vi "Load data into Tree.vi"(8 "error in (no error)":errorcluster, 11 "Execution UI In":refnum<class "Execution UI.lvclass">) -> (0 "error out":errorcluster, 3 "Execution UI Out":refnum<class "Execution UI.lvclass">)   [LabVIEW 2020, in "Execution UI.lvclass"]
uses:
  Execution UI.lvclass
  Execution UI.lvclass/Execution UI.ctl
  Helper Classes/Test Finder/Test Finder.lvclass/Test Finder.ctl
  Helper Classes/Result Table/Result Table/Result Table.lvclass/Result Table.ctl
  Helper Classes/Test Result Tree/Test Result Tree.lvclass
  C:/Users/anton/Documents/GitHub/LUnit/source/Framework/Helper Classes/Test Tree/Test Tree.lvclass
  Helper Classes/Test Finder/Public/Accessors/Read Test Method Names.vi
  Helper Classes/Test Tree/Test Tree.lvclass
  Helper Classes/Test Finder/Test Finder.lvclass
  Helper Classes/Result Table/Result Table/Result Table.lvclass
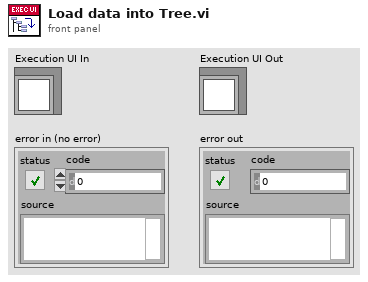
[diagram p1: front panel]
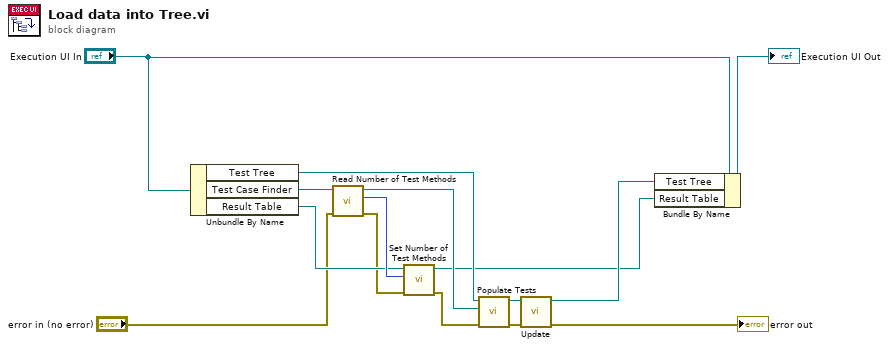
[diagram p0: block diagram]
diagram:
  n1 = Unbundle By Name("Execution UI In") -> ("Test Tree"=w11:refnum<class "Test Result Tree.lvclass">, "Test Case Finder"=w8:refnum<class "Test Finder.lvclass">, "Result Table"=w5:refnum<class "Result Table.lvclass">)
  n2 = call "Read Number of Test Methods.vi"("error in (no error)"="error in (no error)", "Test Finder In"=w8) -> ("error out"=w4:errorcluster, "Number of Test Methods found"=w6:i32, "Test Finder Out"=w7:refnum<class "Test Finder.lvclass">)  [unwired: 7 in]
  n3 = call "Set Number of Test Methods.vi"("error in (no error)"=w4, "Method Count"=w6, "Result Table.lvclass"=w5) -> ("error out"=w2:errorcluster, "Result Table"=w1:refnum<class "Result Table.lvclass">)  [unwired: 7 in]
  n4 = call "Populate Tests.vi"("error in (no error)"=w2, "Test Finder in"=w7, "Test Tree In"=w11) -> ("error out"=w9:errorcluster, "Test Tree Out"=w10:refnum<class "Test Result Tree.lvclass">)  [unwired: 6 in, 1 out]
  n5 = call "Update.vi"("error in (no error)"=w9, "Test Tree In"=w10) -> ("error out"=→"error out":errorcluster, "Test Tree Out"=w12:refnum<class "Test Result Tree.lvclass">)  [unwired: 8 in]
  n6 = Bundle By Name(cluster="Execution UI In", "Test Tree"=w12, "Result Table"=w1) -> (→"Execution UI Out":refnum<class "Execution UI.lvclass">)
